vi "Post-Dig User Hook.vi"(8 "Error In":errorcluster) -> (0 "Error Out":errorcluster)   [LabVIEW 2018, in "Tests.lvlib" / "Toolkit.lvlib" / "Integration.lvlib"]
uses:
  Integration.lvlib
  Support/Hook Search Paths.ctl
  Support/Dig Target.vi
  src/Toolkit/Toolkit.lvlib
  <vilib>/addons/_JKI Toolkits/Caraya/classes/Test/Test.lvclass
  Tests.lvlib
  <vilib>/addons/_JKI Toolkits/Caraya/classes/Assert/Assert.lvclass
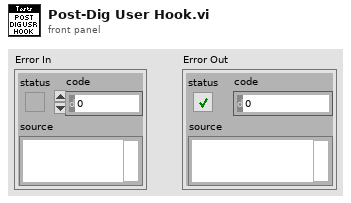
[diagram p1: front panel]
types:
  T1 = typedef "Tests.lvlib/Toolkit.lvlib/Integration.lvlib/Hook Search Paths.ctl" = enum32{"System", "User", "Project (Hidden)", "Project (Visible)"}
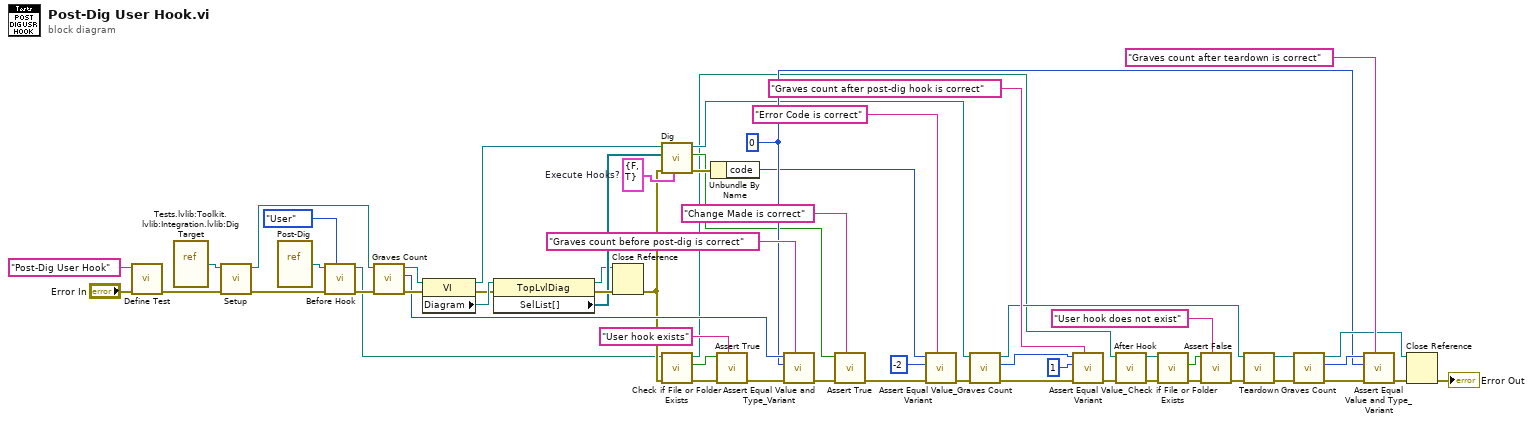
[diagram p0: block diagram]
diagram:
  w29 = cluster{"Pre":bool, "Post":bool} {"Pre"=FALSE, "Post"=TRUE}  # Execute Hooks?
  w33 = 0 ("size(s)")
  n1 = call <vilib>:"Define Test.vi"("error in (no error)"="Error In", "Label (VI Title)"="Post-Dig User Hook") -> ("error out"=w45:errorcluster)  [unwired: 9 in]
  n2 = vi-ref "Tests.lvlib:Toolkit.lvlib:Integration.lvlib:Dig Target.vi"() -> (w30:refnum<vi>)
  n3 = call "Setup.vi"("Error In"=w45, "VI In"=w30) -> ("Error Out"=w17:errorcluster, "VI Out"=w47:refnum<vi>)  [unwired: 8 in]
  n4 = vi-ref "Post-Dig.vi"() -> (w18:refnum<vi>)
  n5 = call "Before Hook.vi"("Hooks Search Path"=Hook_Search_Paths."User", "Error In"=w17, "Hook VI"=w18) -> ("Error Out"=w16:errorcluster, "Hook VI"=w3:path)  [unwired: 7 in]
  n6 = call "Graves Count.vi"("Error In"=w16, "Test Target In"=w47) -> ("Error Out"=w42:errorcluster, "Graves Count"=w41:i32, "Test Target Out"=w46:refnum<vi>)  [unwired: 7 in]
  n7 = property class="VI"(reference=w46, error in=w42) -> (reference out=w55:refnum<vi>, error out=w57:errorcluster, "Diagram"=w58:refnum<vi>)
  n8 = property class="TopLvlDiag"(reference=w58, error in=w57) -> (reference out=w50:refnum<vi>, error out=w56:errorcluster, "SelList[]"=w54:refnum<vi>[])
  n9 = Close Reference(reference=w50, error in (no error)=w56) -> (error out=w5:errorcluster)
  n10 = call "Dig.vi"("Execute Hooks?"=w29, "Error In"=w5, "Selection List"=w54, "VI In"=w55) -> ("Error Out"=w28:errorcluster, "Change Made?"=w21:bool, "VI Out"=w24:refnum<vi>)  [unwired: 5 in]
  n11 = call <vilib>:"Check if File or Folder Exists.vi"("error in (no error)"=w5, "path"=w3) -> ("error out"=w4:errorcluster, "file or folder exists?"=w1:bool, "dup path"=w2:path)  [unwired: 7 in]
  n12 = Unbundle By Name(w28) -> ("code"=w32:i32)
  n13 = call <vilib>:"Assert True.vi"("Label"="User hook exists", "error in (no error)"=w4, "True?"=w1) -> ("error out"=w7:errorcluster)  [unwired: 8 in]
  n14 = call <vilib>:"Assert Equal Value and Type_Variant.vi"("Label"="Graves count before post-dig is correct", "error in (no error)"=w7, "Y"=w33, "X"=w41) -> ("error out"=w44:errorcluster)  [unwired: 7 in]
  n15 = call <vilib>:"Assert True.vi"("Label"="Change Made is correct", "error in (no error)"=w44, "True?"=w21) -> ("error out"=w22:errorcluster)  [unwired: 8 in]
  n16 = call <vilib>:"Assert Equal Value_Variant.vi"("Label"="Error Code is correct", "error in (no error)"=w22, "Y"=-2 ("code"), "X"=w32) -> ("error out"=w27:errorcluster)  [unwired: 7 in]
  n17 = call "Graves Count.vi"("Error In"=w27, "Test Target In"=w24) -> ("Error Out"=w26:errorcluster, "Graves Count"=w25:i32, "Test Target Out"=w23:refnum<vi>)  [unwired: 7 in]
  n18 = call <vilib>:"Assert Equal Value_Variant.vi"("Label"="Graves count after post-dig hook is correct", "error in (no error)"=w26, "Y"=1 ("Graves Count"), "X"=w25) -> ("error out"=w14:errorcluster)  [unwired: 7 in]
  n19 = call "After Hook.vi"("Error In"=w14, "Hook VI In"=w2) -> ("Error Out"=w12:errorcluster, "Hook VI Out"=w13:path)  [unwired: 8 in]
  n20 = call <vilib>:"Check if File or Folder Exists.vi"("error in (no error)"=w12, "path"=w13) -> ("error out"=w10:errorcluster, "file or folder exists?"=w11:bool)  [unwired: 7 in, 1 out]
  n21 = call <vilib>:"Assert False.vi"("Label"="User hook does not exist", "error in (no error)"=w10, "False?"=w11) -> ("error out"=w9:errorcluster)  [unwired: 8 in]
  n22 = call "Teardown.vi"("Error In"=w9, "VI In"=w23) -> ("Error Out"=w36:errorcluster, "VI Out"=w38:refnum<vi>)  [unwired: 8 in]
  n23 = call "Graves Count.vi"("Error In"=w36, "Test Target In"=w38) -> ("Error Out"=w35:errorcluster, "Graves Count"=w34:i32, "Test Target Out"=w37:refnum<vi>)  [unwired: 7 in]
  n24 = call <vilib>:"Assert Equal Value and Type_Variant.vi"("Label"="Graves count after teardown is correct", "error in (no error)"=w35, "Y"=w33, "X"=w34) -> ("error out"=w40:errorcluster)  [unwired: 7 in]
  n25 = Close Reference(reference=w37, error in (no error)=w40) -> (error out=→"Error Out":errorcluster)
